vi "Datasheet Sort Items.vi"(9 "Items":T1[](array[typedef])) -> (1 "Each item tests - Grouped Results":cluster{"Result Group":T1[]}[](array[cluster]))   [LabVIEW 2011]
uses:
  www/cgi-bin/_cgi-lib/TDM_INDEX Record.ctl
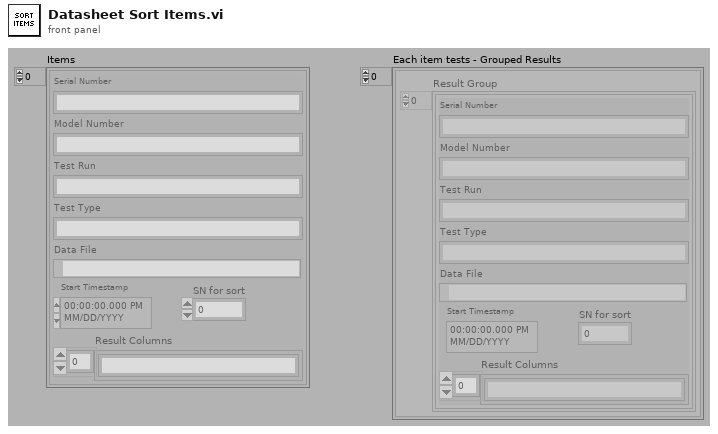
[diagram p1: front panel]
types:
  T1 = typedef "TDM_INDEX Record.ctl" = cluster{"Model Number":string, "SN for sort":i32, "Test Type":string, "Test Run":string, "Serial Number":string, "Start Timestamp":timestamp, "Data File":path, "Result Columns":string[]}
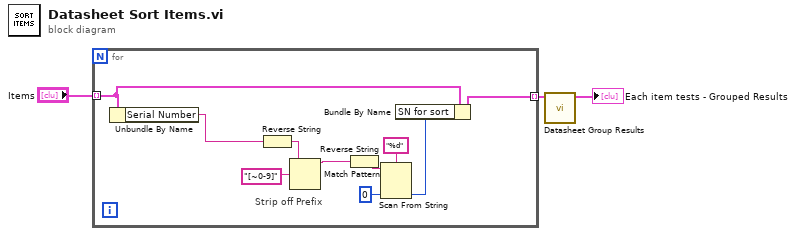
[diagram p0: block diagram]
diagram:
  n1 = for {
    tunnel: "Items" -> [w13] mode=indexing
    tunnel: [w12] -> w1 mode=indexing
    # "Strip off Prefix"
    n2 = Unbundle By Name(w13) -> ("Serial Number"=w4:string)
    n3 = Reverse String(1:w4) -> (0:w9:string)
    n4 = Match Pattern(string=w9, regular expression="[~0-9]" ("format string")) -> (before substring=w11:string)  [unwired: 4 out]
    n5 = Reverse String(1:w11) -> (0:w10:string)
    n6 = Scan From String(format string="%d", input string=w10, default 1=0 ("default value 1")) -> (output 1=w6:i32)  [unwired: 2 in, 3 out]
    n7 = Bundle By Name(cluster=w13, "SN for sort"=w6) -> (w12:T1)
  }
  n8 = call "Datasheet Group Results.vi"("Field Information"=w1) -> ("Each item tests - Grouped Results"=→"Each item tests - Grouped Results":cluster{"Result Group":T1[]}[])  [unwired: 10 out]
